vi "I_Gain.vi"(1 "Shunt Resistor":T1) -> (0 "Gain (V/A)":dbl)   [LabVIEW 2016, in "KH7008.lvclass"]
uses:
  KH7008.lvclass
  typedefs/Shunt-Enum.ctl
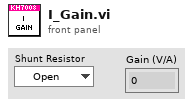
[diagram p1: front panel]
types:
  T1 = typedef "KH7008.lvclass/Shunt-Enum.ctl" = enum16{"Open", "50 Ohms", "500 Ohms", "5k Ohms", "50k Ohms"}
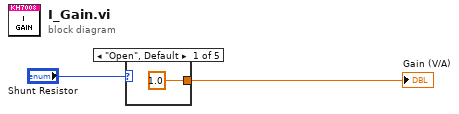
[diagram p0: block diagram]
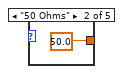
[diagram p2: hidden frame]
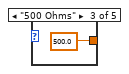
[diagram p3: hidden frame]
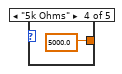
[diagram p4: hidden frame]
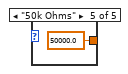
[diagram p5: hidden frame]
diagram:
  n1 = case shown="\"Open\", Default" "Shunt Resistor" {
    tunnel: [1.0 ("y") 50.0 ("y") 500.0 ("y") 5000.0 ("y") 50000.0 ("y")] -> w2
    frame "Open", Default {
    }
    frame "50 Ohms" {
    }
    frame "500 Ohms" {
    }
    frame "5k Ohms" {
    }
    frame "50k Ohms" {
    }
  }
  "Gain (V/A)" <- w2
